vi "Destory.vi"(8 "error in (no error)":errorcluster, 11 "DataContainer in":refnum<class "DataContainer.lvclass">) -> (0 "error out":errorcluster, 3 "DataContainer out":refnum<class "DataContainer.lvclass">)   [LabVIEW 2023, in "DataContainer.lvclass"]
uses:
  DataContainer.lvclass
  DataContainer.lvclass/DataContainer.ctl
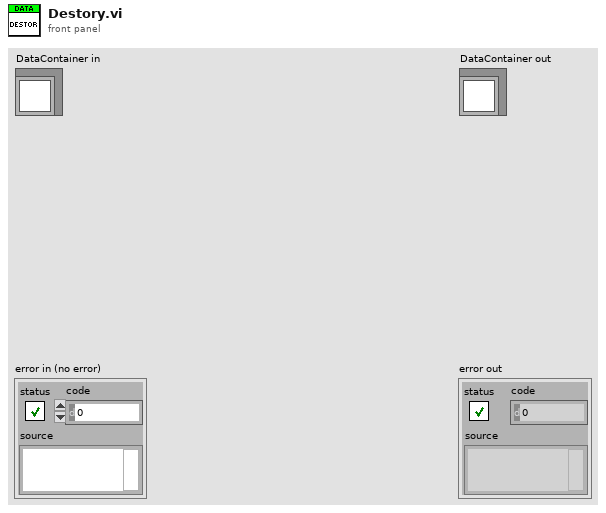
[diagram p1: front panel]
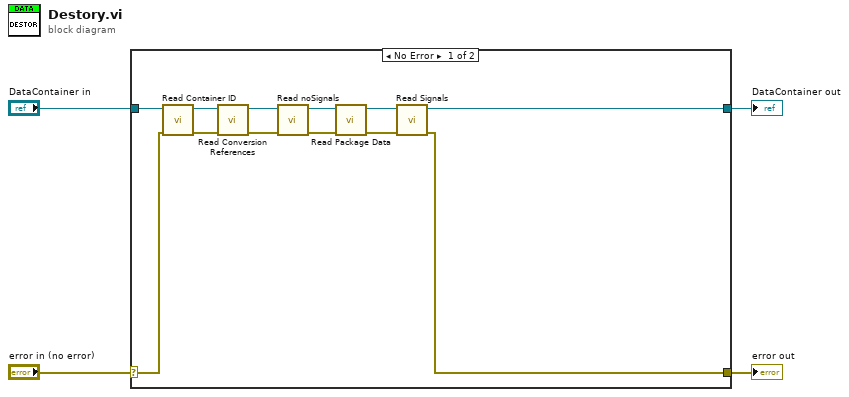
[diagram p0: block diagram]
diagram:
  n1 = case shown="No Error" "error in (no error)" {
    selector: "error in (no error)" -> [w6 w18]
    tunnel: [w5 w18] -> w3
    tunnel: [w7 w17] -> w1
    tunnel: "DataContainer in" -> [w8 w17]
    frame No Error {
      n2 = call-dynamic "Read Container ID.vi"("error in (no error)"=w6, "DataContainer in"=w8) -> ("error out"=w15:errorcluster, "DataContainer out"=w16:refnum<class "DataContainer.lvclass">)  [unwired: 7 in, 1 out]
      n3 = call-dynamic "Read Conversion References.vi"("error in (no error)"=w15, "DataContainer in"=w16) -> ("error out"=w13:errorcluster, "DataContainer out"=w14:refnum<class "DataContainer.lvclass">)  [unwired: 7 in, 1 out]
      n4 = call-dynamic "Read noSignals.vi"("error in (no error)"=w13, "DataContainer in"=w14) -> ("error out"=w11:errorcluster, "DataContainer out"=w12:refnum<class "DataContainer.lvclass">)  [unwired: 7 in, 1 out]
      n5 = call-dynamic "Read Package Data.vi"("error in (no error)"=w11, "DataContainer in"=w12) -> ("error out"=w9:errorcluster, "DataContainer out"=w10:refnum<class "DataContainer.lvclass">)  [unwired: 7 in, 1 out]
      n6 = call-dynamic "Read Signals.vi"("error in (no error)"=w9, "DataContainer in"=w10) -> ("error out"=w5:errorcluster, "DataContainer out"=w7:refnum<class "DataContainer.lvclass">)  [unwired: 7 in, 1 out]
    }
    frame Error {
    }
  }
  "error out" <- w3
  "DataContainer out" <- w1
